vi "Run.vi"(6 "Type y_pred":T1(ring), 7 "Type y_true":T1(ring), 8 "error in (no error)":errorcluster caption="entrée d'erreur (pas d'erreur)", 9 "y_pred":string[][](array[string]), 10 "y_true":string[][](array[string]), 11 "Classification_Report.lvclass":refnum<class "Classification_Report.lvclass">) -> (0 "error out":errorcluster caption="sortie d'erreur", 2 "String Data":string, 3 "Classification_Report.lvclass":refnum<class "Classification_Report.lvclass">)   [LabVIEW 2020, in "Classification_Report.lvclass"]
doc: "Returns :\n\n- report : string / dict\nText summary of the precision, recall, F1 score for each class. Dictionary returned if output_dict is True. Dictionary has the following structure:\n\n{'label 1': {'precision':0.5,\n 'recall':1.0,\n 'f1-score':0.67,\n 'support':1},\n 'label 2': { ... },\n ...\n}\n\nThe reported averages include macro average (averaging the unweighted mean per label), weighted average (averaging the support-weighted mean per label), and sample average (only for multilabel classification). Micro average (averaging the total true positives, false negatives and false positives) is only shown for multi-label or multi-class with a subset of classes, because it corresponds to accuracy otherwise. See also precision_recall_fscore_support for more details on averages.\n\nNote that in binary classification, recall of the positive class is also known as “sensitivity”; recall of the negative class is “specificity”."
uses:
  Classification_Report.lvclass
  Classification_Report.lvclass/Classification_Report.ctl
panel:
  in  "Type y_pred":T1(ring)
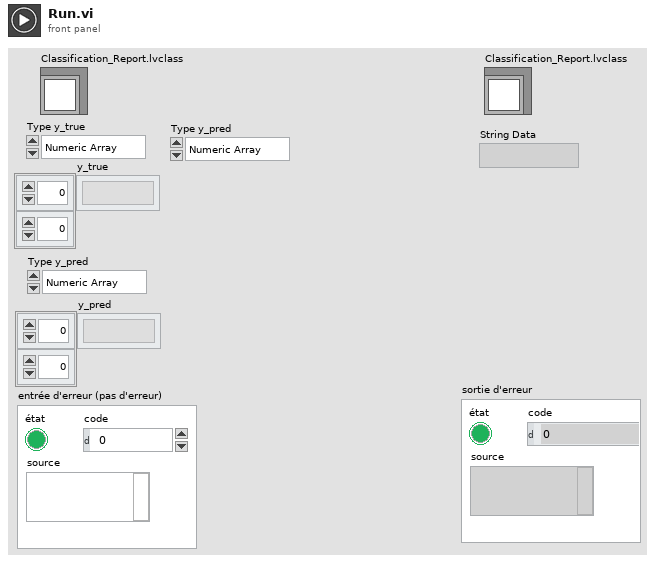
[diagram p1: front panel]
types:
  T1 = enum16{"Numeric Array", "String Array", "Sparse"}
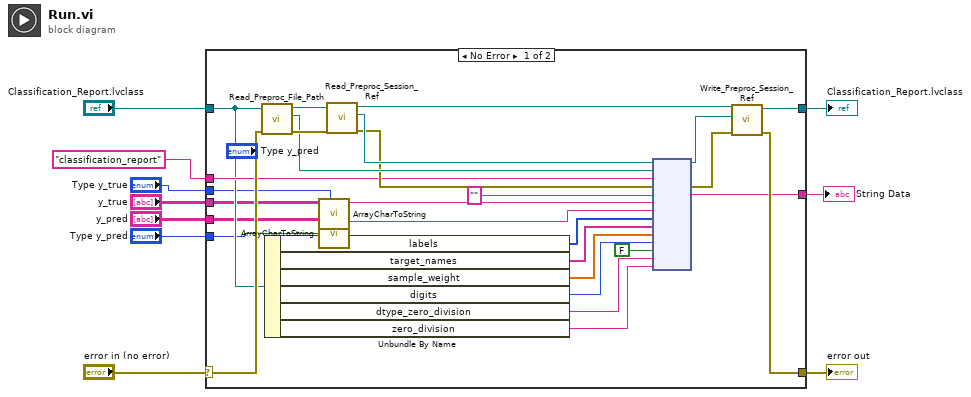
[diagram p0: block diagram]
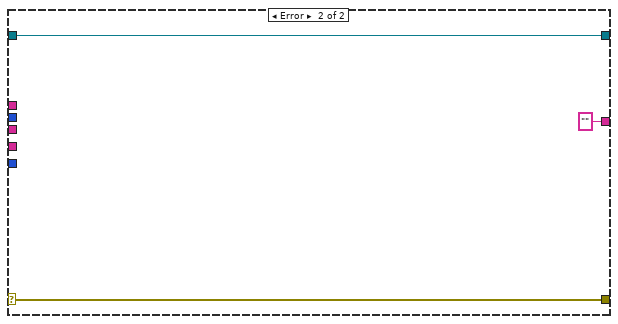
[diagram p2: hidden frame]
diagram:
  n1 = case shown="No Error" "error in (no error)" {
    selector: "error in (no error)" -> [w27 w41]
    tunnel: [w28 w41] -> w9
    tunnel: [w29 w40] -> w7
    tunnel: "Classification_Report.lvclass" -> [w24 w40]
    tunnel: "classification_report" -> [w26 _]
    tunnel: [w25 ""] -> w6
    tunnel: "y_true" -> [w16 _]
    tunnel: "y_pred" -> [w15 _]
    tunnel: "Type y_true" -> [w12 _]
    tunnel: "Type y_pred" -> [w11 _]
    frame No Error {
      n2 = call-dynamic "Read_Preproc_File_Path.vi"("error in (no error)"=w27, "Python in"=w24) -> ("error out"=w37:errorcluster, "File_Path"=w36:path, "Python out"=w38:refnum<class "Classification_Report.lvclass">)  [unwired: 7 in]
      n3 = Unbundle By Name(w24) -> ("labels"=w23:i32[], "target_names"=w22:string[], "sample_weight"=w21:dbl[], "digits"=w20:i32, "dtype_zero_division"=w18:string, "zero_division"=w17:string)
      n4 = call "ArrayCharToString.vi"("Type"=w12, "TAB"=w16) -> ("Instruction"=w13:string)  [unwired: 9 in]
      n5 = call "ArrayCharToString.vi"("Type"=w11, "TAB"=w15) -> ("Instruction"=w14:string)  [unwired: 9 in]
      n6 = call-dynamic "Read_Preproc_Session_Ref.vi"("error in (no error)"=w37, "Python in"=w38) -> ("error out"=w34:errorcluster, "Session_ref"=w35:refnum<k35>, "Python out"=w33:refnum<class "Classification_Report.lvclass">)  [unwired: 7 in]
      n7 = node(w35, w36, w26, w34, "", w13, w14, w23, w22, w21, w20, FALSE, w18, w17) -> (w31:refnum<k35>, w32:errorcluster, w25:string)  [unwired: 9 in, 2 out]
      n8 = call-dynamic "Write_Preproc_Session_Ref.vi"("error in (no error)"=w32, "Session_ref"=w31, "Python in"=w33) -> ("error out"=w28:errorcluster, "Python out"=w29:refnum<class "Classification_Report.lvclass">)  [unwired: 7 in]
    }
    frame Error {
    }
  }
  "error out" <- w9
  "Classification_Report.lvclass" <- w7
  "String Data" <- w6
